vi "CRYView Part Load VI.vi"(8 "sData":string, 11 "sAction":string) -> (1 "tWindow_Out":T1)   [LabVIEW 2013]
uses:
  CRYView Global.vi
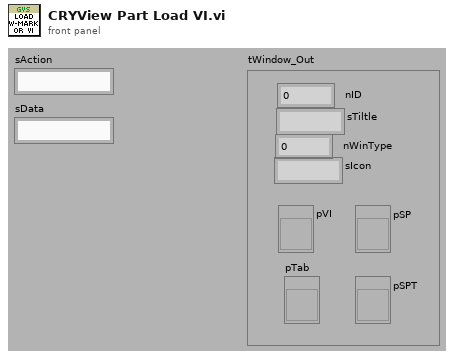
[diagram p1: front panel]
types:
  T1 = cluster{"nID":i32, "sTiltle":string, "pVI":refnum<vi>, "pSP":refnum<vi>, "pTab":refnum<vi>, "pSPT":refnum<vi>, "nWinType":i32, "sIcon":string}
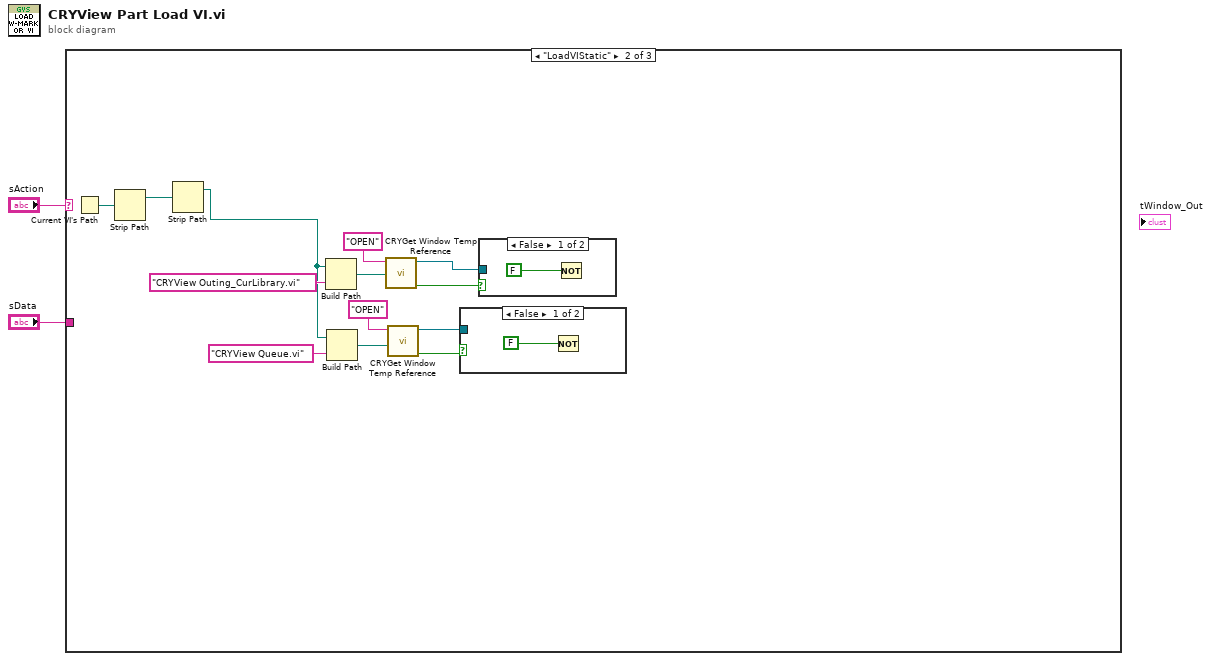
[diagram p0: block diagram]
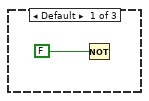
[diagram p2: hidden frame]
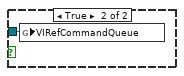
[diagram p3: hidden frame]
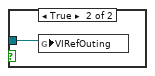
[diagram p4: hidden frame]
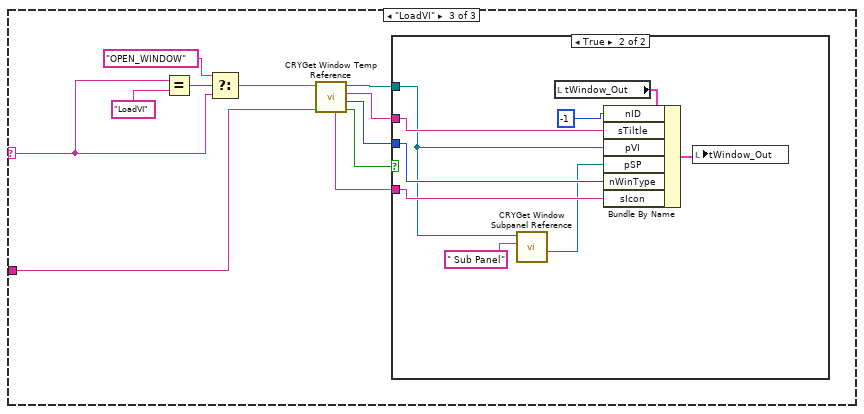
[diagram p5: hidden frame]
diagram:
  n1 = case shown="\"LoadVIStatic\"" "sAction" {
    selector: "sAction" -> [_ _ w22]
    tunnel: "sData" -> [_ _ w27]
    frame Default {
      n2 = Not(x=FALSE) -> ()  [unwired: 1 out]
    }
    frame "LoadVIStatic" {
      n3 = Current VI's Path() -> (path=w16:path)
      n4 = Strip Path(path=w16) -> (stripped path=w5:path)  [unwired: 1 out]
      n5 = Strip Path(path=w5) -> (stripped path=w4:path)  [unwired: 1 out]
      n6 = Build Path(base path=w4, name or relative path="CRYView Outing_CurLibrary.vi") -> (appended path=w15:path)
      n7 = Build Path(base path=w4, name or relative path="CRYView Queue.vi") -> (appended path=w9:path)
      n8 = call "CRYGet Window Temp Reference.vi"("sVIFullName"=w15, "sAction"="OPEN") -> ("bResult"=w13:bool, "pVIRef_Out"=w12:refnum<vi>)  [unwired: 5 in, 3 out]
      n9 = call "CRYGet Window Temp Reference.vi"("sVIFullName"=w9, "sAction"="OPEN") -> ("bResult"=w6:bool, "pVIRef_Out"=w8:refnum<vi>)  [unwired: 5 in, 3 out]
      n10 = case shown="False" w6 {
        tunnel: w8 -> [_ w18]
        frame False {
          n11 = Not(x=FALSE) -> ()  [unwired: 1 out]
        }
        frame True {
          n12 = global write "CRYView Global.vi" "VIRefCommandQueue"(w18) -> ()
        }
      }
      n13 = case shown="False" w13 {
        tunnel: w12 -> [_ w20]
        frame False {
          n14 = Not(x=FALSE) -> ()  [unwired: 1 out]
        }
        frame True {
          n15 = global write "CRYView Global.vi" "VIRefOuting"(w20) -> ()
        }
      }
    }
    frame "LoadVI" {
      n16 = Equal?(x=w22, y="LoadVI" ("sAction")) -> (x = y?=w24:bool)
      n17 = Select(t="OPEN_WINDOW" ("sAction"), s=w24, f=w22) -> (s? t:f=w21:string)
      n18 = call "CRYGet Window Temp Reference.vi"("sWindowName"=w27, "sAction"=w21) -> ("bResult"=w29:bool, "nWinType"=w31:i32, "sTitleName Out"=w30:string, "pVIRef_Out"=w28:refnum<vi>, "sIcon_Out"=w26:string)  [unwired: 5 in]
      n19 = case shown="True" w29 {
        tunnel: w28 -> [_ w34]
        tunnel: w30 -> [_ w39]
        tunnel: w31 -> [_ w37]
        tunnel: w26 -> [_ w36]
        frame False {
        }
        frame True {
          n20 = call "CRYGet Window Subpanel Reference.vi"("Sub Panel Name"=" Sub Panel", "VI Ref In"=w34) -> ("SubPnl Refnum"=w33:refnum<vi>)  [unwired: 7 in, 2 out]
          n21 = local read "tWindow_Out"() -> (w35:T1)
          n22 = Bundle By Name(cluster=w35, "nID"=-1, "sTiltle"=w39, "pVI"=w34, "pSP"=w33, "nWinType"=w37, "sIcon"=w36) -> (w38:T1)
          n23 = local write "tWindow_Out"(w38) -> ()
        }
      }
    }
  }
